vi "Edit Wet Cryo.vi"(8 "error in":errorcluster, 11 "Instrument parameters in":T1) -> (0 "error out":errorcluster, 3 "Instrument parameters out":T1)   [LabVIEW 2025]
uses:
  Cryo.lvlib
panel:
  in  "stop":bool
  out "error status":errorcluster
  in  "Polling time\n offset":i32
  in  "Wait time\nbefore hold (ms)":i32
  in  "Precision 2":dbl=0.0001 caption="Precision"
  in  "Initialize cryo magnet?":bool
  # "Settings for wet cryostat..."
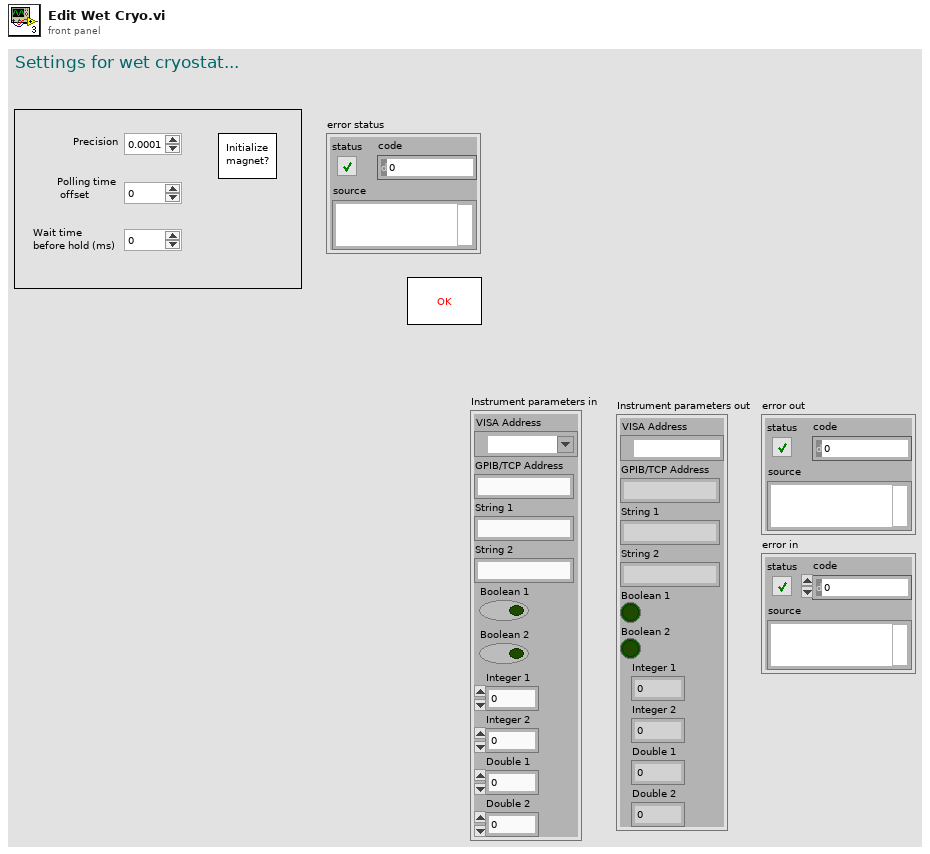
[diagram p1: front panel]
types:
  T1 = cluster{"VISA Address":refnum<visa-resource-name>, "GPIB/TCP Address":string, "String 1":string, "String 2":string, "Boolean 1":bool, "Boolean 2":bool, "Integer 1":i32, "Integer 2":i32, "Double 1":dbl, "Double 2":dbl}
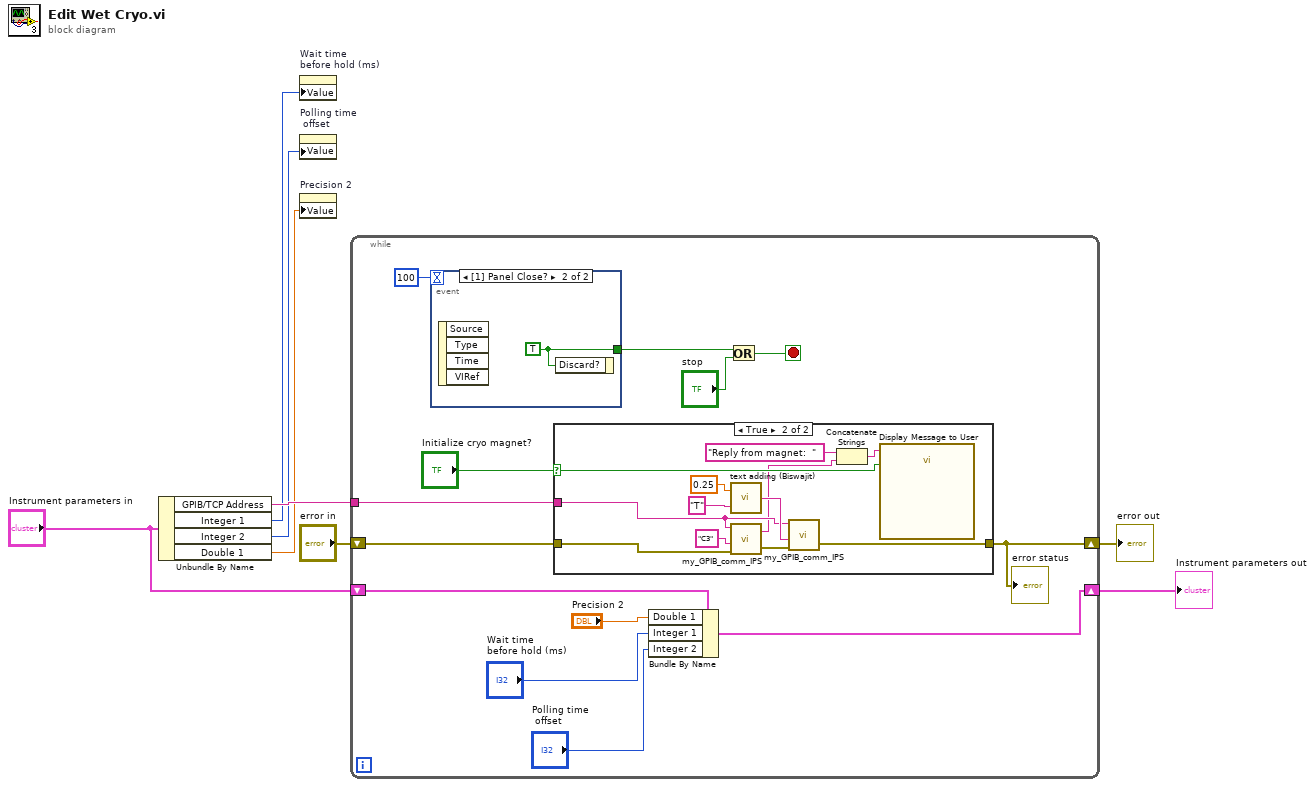
[diagram p0: block diagram]
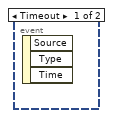
[diagram p3: hidden frame]
diagram:
  n1 = Unbundle By Name("Instrument parameters in") -> ("GPIB/TCP Address"=w4:string, "Integer 1"=w3:i32, "Integer 2"=w2:i32, "Double 1"=w1:dbl)
  n2 = property on="Wait time\nbefore hold (ms)" class="DigNum (strict)"("Value"=w3) -> ()  [unwired: 2 in, 2 out]
  n3 = property on="Polling time\n offset" class="DigNum (strict)"("Value"=w2) -> ()  [unwired: 2 in, 2 out]
  n4 = property on="Precision 2" class="DigNum (strict)"("Value"=w1) -> ()  [unwired: 2 in, 2 out]
  n5 = while {
    shift-right: [w16] -> w8
    shift-left: "Instrument parameters in" -> [w18]
    shift-right: [w12] -> w6
    shift-left: "error in" -> [w20]
    tunnel: w4 -> [w13]
    stop <- w9 stop-if-true
    n6 = event shown="[1] Panel Close?" {
      selector: _ -> [_ _]
      dyn-events: _ -> [_ _]
      timeout: 100 -> [_ _]
      tunnel: [_ w35] -> w11
      event Timeout {
        n7 = event-data() -> ()  [unwired: 1 in, 3 out]
      }
      event Panel Close? {
        w35 = TRUE ("Discard?")
        n8 = event-data() -> ()  [unwired: 1 in, 4 out]
        n9 = event-data("Discard?"=w35) -> ()  [unwired: 1 in, 1 out]
      }
    }
    n10 = case shown="True" "Initialize cryo magnet?" {
      selector: "Initialize cryo magnet?" -> [_ w26]
      tunnel: w20 -> [w22 w30]
      tunnel: [w22 w28] -> w12
      tunnel: w13 -> [_ w27]
      frame False {
      }
      frame True {
        n11 = call "text adding (Biswajit).vi"("string"="T", "number"=0.25 ("Sweep rate (T/min)")) -> ("String"=w33:string)
        n12 = call "my_GPIB_comm_IPS.vi"("error in"=w30, "Command"="C3", "GPIB address"=w27) -> ("error out"=w29:errorcluster, "Reply from Instrument"=w25:string)  [unwired: 1 in]
        n13 = call "my_GPIB_comm_IPS.vi"("error in"=w29, "Command"=w33, "GPIB address"=w27) -> ("error out"=w28:errorcluster)  [unwired: 1 in, 1 out]
        n14 = Concatenate Strings("Reply from magnet:  " ("string"), w25) -> (w24:string)
        n15 = call "Display Message to User"("Enable"=w26, "Message"=w24) -> ()  [unwired: 8 in, 2 out]
      }
    }
    "error status" <- w12
    n16 = Bundle By Name(cluster=w18, "Double 1"="Precision 2", "Integer 1"="Wait time\nbefore hold (ms)", "Integer 2"="Polling time\n offset") -> (w16:T1)
    n17 = Or(x=w11, y="stop") -> (x .or. y?=w9:bool)
  }
  "Instrument parameters out" <- w8
  "error out" <- w6
